vi "Session.CheckValid.vi"(10 "Cached Session":T1, 11 "requested session":T1) -> (2 "Error Code":i32, 3 "Valid?":bool)   [LabVIEW 2025, in "xnet_can_bus_monitor_api_server_do.lvlib"]
uses:
  xnet_can_bus_monitor_api_server_do.lvlib
  xnet_can_bus_monitor_api_server/RPC Messages/ni_xnet_can_bm_api_Session.ctl
  xnet_can_bus_monitor_api_server/xnet_can_bus_monitor_api_server.lvlib
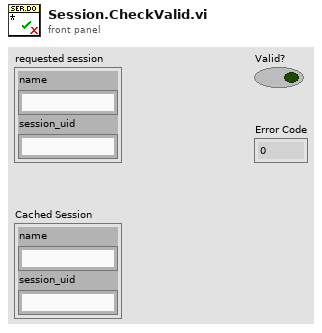
[diagram p1: front panel]
types:
  T1 = typedef "xnet_can_bus_monitor_api_server.lvlib/ni_xnet_can_bm_api_Session.ctl" = cluster{"name":string, "session_uid":string}
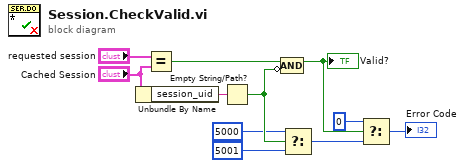
[diagram p0: block diagram]
diagram:
  n1 = Unbundle By Name("Cached Session") -> ("session_uid"=w8:string)
  n2 = Equal?(x="requested session", y="Cached Session") -> (x = y?=w11:bool)
  n3 = Empty String/Path?(string/path=w8) -> (empty?=w7:bool)
  n4 = Compound Arithmetic op=AND(w11, invert w7) -> (w4:bool)
  "Valid?" <- w4
  n5 = Select(t=5000 ("error code (0)"), s=w7, f=5001 ("error code (0)")) -> (s? t:f=w3:i32)
  n6 = Select(t=0, s=w4, f=w3) -> (s? t:f=→"Error Code":i32)
